vi "DistanciaPuntos.vi"() -> ()   [LabVIEW 2018]
panel:
  in  "Y2":dbl
  out "DISTANCIA":dbl
  in  "X2":dbl
  in  "Y1":dbl
  in  "X1":dbl
  # "PUNTOS"
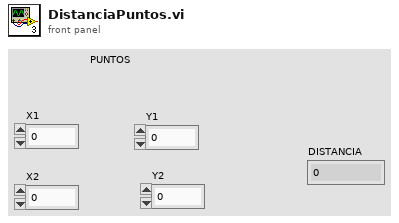
[diagram p1: front panel]
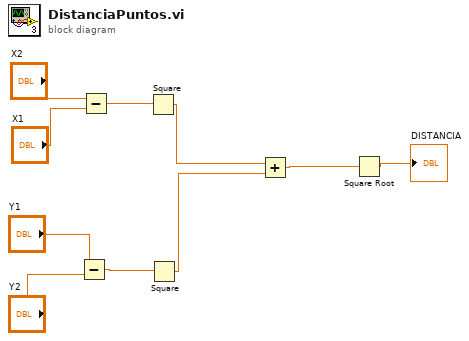
[diagram p0: block diagram]
diagram:
  n1 = Subtract(x="Y1", y="Y2") -> (x-y=w5:dbl)
  n2 = Subtract(x="X2", y="X1") -> (x-y=w6:dbl)
  n3 = Square(x=w6) -> (x^2=w8:dbl)
  n4 = Square(x=w5) -> (x^2=w7:dbl)
  n5 = Add(x=w8, y=w7) -> (x+y=w9:dbl)
  n6 = Square Root(x=w9) -> (sqrt(x)=→"DISTANCIA":dbl)
